vi "Get stack field.vi"(7 "Is Module?":bool, 8 "error in (no error)":errorcluster, 10 "Field":string, 11 "Stack in":refnum<class "Stack.lvclass">) -> (0 "error out":errorcluster, 1 "Value out":string, 3 "Stack out":refnum<class "Stack.lvclass">)   [LabVIEW 2022 SP3, in "Stack.lvclass"]
uses:
  Stack.lvclass
  Stack.lvclass/Stack.ctl
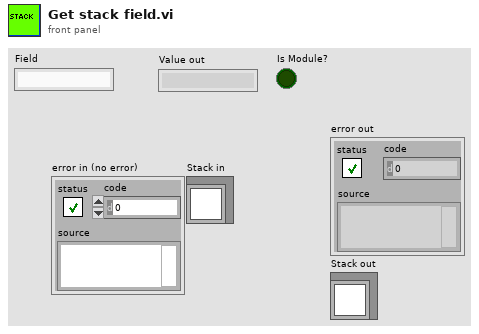
[diagram p1: front panel]
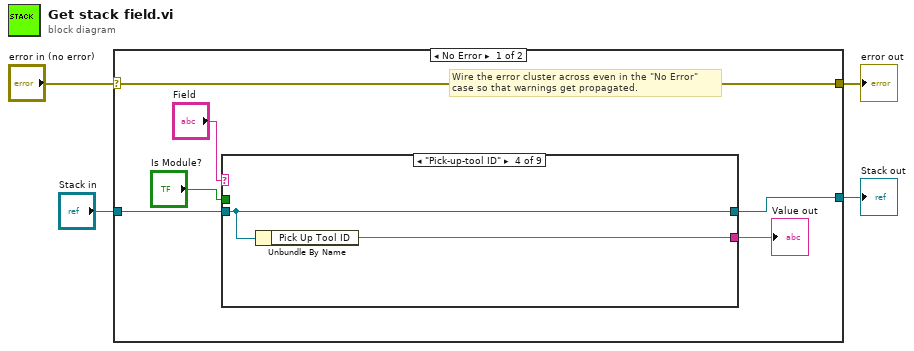
[diagram p0: block diagram]
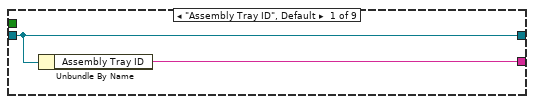
[diagram p2: hidden frame]
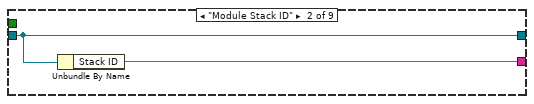
[diagram p3: hidden frame]
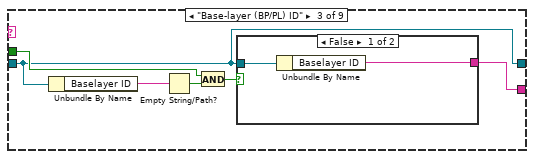
[diagram p4: hidden frame]
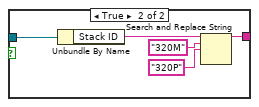
[diagram p5: hidden frame]
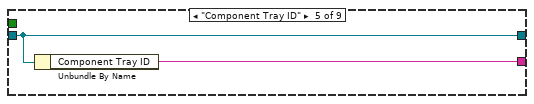
[diagram p6: hidden frame]
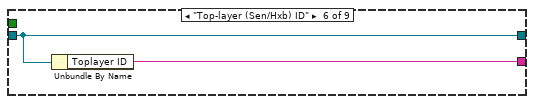
[diagram p7: hidden frame]
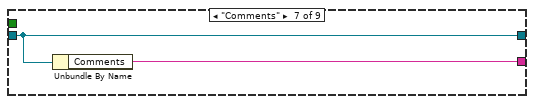
[diagram p8: hidden frame]
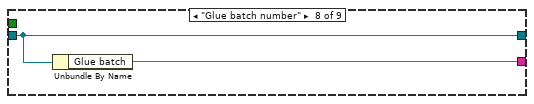
[diagram p9: hidden frame]
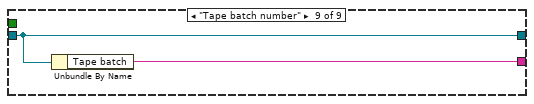
[diagram p10: hidden frame]
diagram:
  n1 = case shown="No Error" "error in (no error)" {
    selector: "error in (no error)" -> [w10 w41]
    tunnel: [w10 w41] -> w3
    tunnel: [w8 w40] -> w1
    tunnel: "Stack in" -> [w9 w40]
    frame No Error {
      # "Wire the error cluster across even in the \"No Error\"\ncase so that warnings get propagated."
      n2 = case shown="\"Pick-up-tool ID\"" "Field" {
        tunnel: w9 -> [w12 w13 w15 w29 w31 w33 w35 w37 w39]
        tunnel: [w12 w13 w15 w29 w31 w33 w35 w37 w39] -> w8
        tunnel: [w11 w14 w20 w28 w30 w32 w34 w36 w38] -> w6
        tunnel: "Is Module?" -> [_ _ w18 _ _ _ _ _ _]
        frame "Assembly Tray ID", Default {
          n3 = Unbundle By Name(w12) -> ("Assembly Tray ID"=w11:string)
        }
        frame "Module Stack ID" {
          n4 = Unbundle By Name(w13) -> ("Stack ID"=w14:string)
        }
        frame "Base-layer (BP/PL) ID" {
          n5 = Unbundle By Name(w15) -> ("Baselayer ID"=w19:string)
          n6 = Empty String/Path?(string/path=w19) -> (empty?=w17:bool)
          n7 = And(x=w18, y=w17) -> (x .and. y?=w16:bool)
          n8 = case shown="False" w16 {
            tunnel: [w22 w25] -> w20
            tunnel: w15 -> [w21 w24]
            frame False {
              n9 = Unbundle By Name(w21) -> ("Baselayer ID"=w22:string)
            }
            frame True {
              n10 = Unbundle By Name(w24) -> ("Stack ID"=w23:string)
              n11 = Search and Replace String(input string=w23, search string="320M", replace string="320P" ("replace string (\"\")")) -> (result string=w25:string)  [unwired: 5 in, 3 out]
            }
          }
        }
        frame "Pick-up-tool ID" {
          n12 = Unbundle By Name(w29) -> ("Pick Up Tool ID"=w28:string)
        }
        frame "Component Tray ID" {
          n13 = Unbundle By Name(w31) -> ("Component Tray ID"=w30:string)
        }
        frame "Top-layer (Sen/Hxb) ID" {
          n14 = Unbundle By Name(w33) -> ("Toplayer ID"=w32:string)
        }
        frame "Comments" {
          n15 = Unbundle By Name(w35) -> ("Comments"=w34:string)
        }
        frame "Glue batch number" {
          n16 = Unbundle By Name(w37) -> ("Glue batch"=w36:string)
        }
        frame "Tape batch number" {
          n17 = Unbundle By Name(w39) -> ("Tape batch"=w38:string)
        }
      }
      "Value out" <- w6
    }
    frame Error {
    }
  }
  "error out" <- w3
  "Stack out" <- w1
